vi "Send Global Chat.vi"(8 "error in (no error)":errorcluster, 10 "Message":string, 11 "Server in":refnum<class "Server.lvclass">) -> (0 "error out":errorcluster, 3 "Server out":refnum<class "Server.lvclass">)   [LabVIEW 2015, in "Server.lvlib" / "Server.lvclass"]
uses:
  Server.lvclass
  Chat Window Model/Chat Window Model Messages/New Message Msg/New Message Msg.lvclass
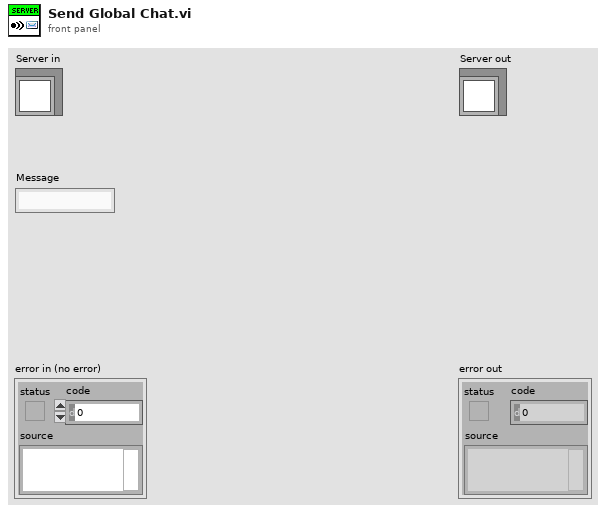
[diagram p1: front panel]
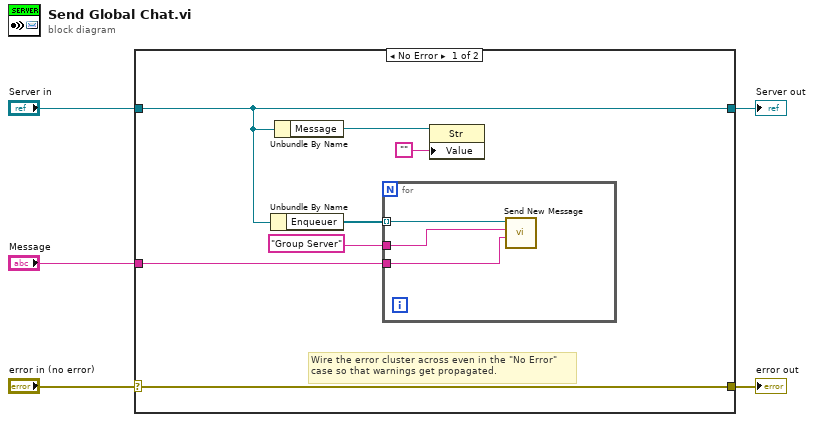
[diagram p0: block diagram]
diagram:
  n1 = case shown="No Error" "error in (no error)" {
    selector: "error in (no error)" -> [w12 w17]
    tunnel: [w12 w17] -> w4
    tunnel: [w8 w16] -> w2
    tunnel: "Server in" -> [w8 w16]
    tunnel: "Message" -> [w11 _]
    frame No Error {
      # "Wire the error cluster across even in the \"No Error\"\ncase so that warnings get propagated."
      n2 = Unbundle By Name(w8) -> ("Enqueuer"=w9:refnum<class "Message Enqueuer.lvclass">[])
      n3 = Unbundle By Name(w8) -> ("Message"=w7:refnum<vi>)
      n4 = for {
        tunnel: w9 -> [w15] mode=indexing
        tunnel: w11 -> [w14]
        tunnel: "Group Server" -> [w13]
        n5 = call "Send New Message.vi"("New Message"=w14, "From"=w13, "Message Enqueuer"=w15) -> ()  [unwired: 7 in, 2 out]
      }
      n6 = property class="Str"(reference=w7, "Value"="") -> ()  [unwired: 1 in, 2 out]
    }
    frame Error {
    }
  }
  "error out" <- w4
  "Server out" <- w2
